vi "VI Tree.vi"   [LabVIEW 2020, in "ChromTech MX-Class Drivers.lvlib"]
doc: "This is the instrument driver for the <INSTRUMENT NAME>. The VI Tree displays all the user-callable VIs of the instrument driver in an organized table."
uses:
  <instrlib>/RxnRover/ChromtechNextGenDriver/ChromTech MX-Class Drivers.lvlib
panel:
  # "(c) 2014 <Enter Company Name Here>.  ALL RIGHTS RESERVED."
  # "SEE DIAGRAM\nFOR VI TREE."
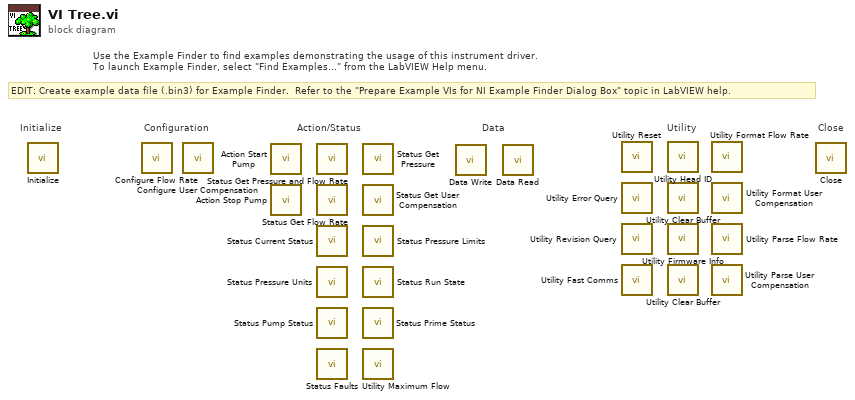
[diagram p0: block diagram]
diagram:
  # "EDIT: Create example data file (.bin3) for Example Finder.  Refer to the \"Prepare Example VIs for NI Example Finder Dialog Box\" topic in LabVIEW help."
  # "Use the Example Finder to find examples demonstrating the usage of this instrument driver.\nTo launch Example Finder, select \"Find Examples...\" from the LabVIEW Help menu."
  # "Configuration"
  # "Utility"
  # "Data"
  # "Action/Status"
  # "Close"
  # "Initialize"
  n1 = call <instrlib>:"Initialize.vi"() -> ()  [unwired: 10 in, 2 out]
  n2 = call <instrlib>:"Configure Flow Rate.vi"() -> ()  [unwired: 9 in, 3 out]
  n3 = call <instrlib>:"Configure User Compensation.vi"() -> ()  [unwired: 3 in, 3 out]
  n4 = call <instrlib>:"Action Start Pump.vi"() -> ()  [unwired: 10 in, 2 out]
  n5 = call <instrlib>:"Action Stop Pump.vi"() -> ()  [unwired: 10 in, 2 out]
  n6 = call <instrlib>:"Status Get Pressure and Flow Rate.vi"() -> ()  [unwired: 8 in, 4 out]
  n7 = call <instrlib>:"Status Get Flow Rate.vi"() -> ()  [unwired: 9 in, 3 out]
  n8 = call <instrlib>:"Status Current Status.vi"() -> ()  [unwired: 9 in, 3 out]
  n9 = call <instrlib>:"Status Pressure Units.vi"() -> ()  [unwired: 9 in, 3 out]
  n10 = call <instrlib>:"Status Pump Status.vi"() -> ()  [unwired: 9 in, 3 out]
  n11 = call <instrlib>:"Status Faults.vi"() -> ()  [unwired: 11 in, 5 out]
  n12 = call <instrlib>:"Status Get Pressure.vi"() -> ()  [unwired: 9 in, 3 out]
  n13 = call <instrlib>:"Status Get User Compensation.vi"() -> ()  [unwired: 3 in, 3 out]
  n14 = call <instrlib>:"Status Pressure Limits.vi"() -> ()  [unwired: 8 in, 4 out]
  n15 = call <instrlib>:"Status Run State.vi"() -> ()  [unwired: 9 in, 3 out]
  n16 = call <instrlib>:"Status Prime Status.vi"() -> ()  [unwired: 9 in, 3 out]
  n17 = call <instrlib>:"Utility Maximum Flow.vi"() -> ()  [unwired: 3 in, 3 out]
  n18 = call <instrlib>:"Data Write.vi"() -> ()  [unwired: 10 in, 2 out]
  n19 = call <instrlib>:"Data Read.vi"() -> ()  [unwired: 9 in, 3 out]
  n20 = call <instrlib>:"Utility Reset.vi"() -> ()  [unwired: 10 in, 2 out]
  n21 = call <instrlib>:"Utility Error Query.vi"() -> ()  [unwired: 8 in, 4 out]
  n22 = call <instrlib>:"Utility Revision Query.vi"() -> ()  [unwired: 8 in, 4 out]
  n23 = call <instrlib>:"Utility Fast Comms.vi"() -> ()  [unwired: 11 in, 1 out]
  n24 = call <instrlib>:"Utility Head ID.vi"() -> ()  [unwired: 9 in, 3 out]
  n25 = call <instrlib>:"Utility Clear Buffer.vi"() -> ()  [unwired: 10 in, 2 out]
  n26 = call <instrlib>:"Utility Firmware Info.vi"() -> ()  [unwired: 8 in, 4 out]
  n27 = call <instrlib>:"Utility Clear Buffer.vi"() -> ()  [unwired: 10 in, 2 out]
  n28 = call <instrlib>:"Utility Format Flow Rate.vi"() -> ()  [unwired: 10 in, 2 out]
  n29 = call <instrlib>:"Utility Format User Compensation.vi"() -> ()  [unwired: 10 in, 2 out]
  n30 = call <instrlib>:"Utility Parse Flow Rate.vi"() -> ()  [unwired: 10 in, 2 out]
  n31 = call <instrlib>:"Utility Parse User Compensation.vi"() -> ()  [unwired: 10 in, 2 out]
  n32 = call <instrlib>:"Close.vi"() -> ()  [unwired: 11 in, 1 out]
